vi "Valves_Widefield.vi"(1 "All Off?":bool, 2 "valve#":i32) -> ()   [LabVIEW 2012]
uses:
  <vilib>/DAQmx/create/channels.llb/DAQmx Create Channel (DO-Digital Output).vi
  <vilib>/DAQmx/write.llb/DAQmx Write (Digital 1D Bool NChan 1Samp 1Line).vi
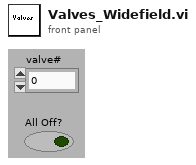
[diagram p1: front panel]
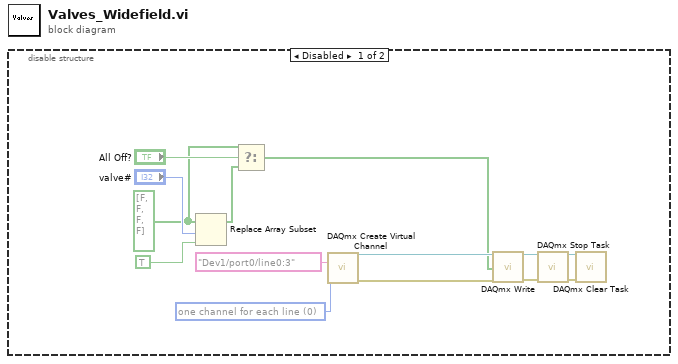
[diagram p0: block diagram]
diagram:
  n1 = disable-structure shown="Disabled" {
    frame Disabled {
      w3 = bool[] [FALSE, FALSE, FALSE, FALSE] ("port status")
      w7 = 0 items=["one channel for each line", "one channel for all lines"] ("line grouping")
      n2 = Replace Array Subset(array=w3, new element=TRUE ("new element/subarray"), index="valve#") -> (w2:bool[])
      n3 = Select(t=w3, s="All Off?", f=w2) -> (s? t:f=w1:bool[])
      n4 = call-poly <vilib>:"DAQmx Create Virtual Channel.vi"("lines"=tag "Dev1/port0/line0:3", "line grouping"=w7) -> ("task out"=w13:refnum<k21>, "error out"=w12:errorcluster)  [unwired: 3 in, 9 out]
      n5 = call-poly <vilib>:"DAQmx Write.vi"("task/channels in"=w13, "data"=w1, "error in"=w12) -> ("task out"=w11:refnum<k21>, "error out"=w10:errorcluster)  [unwired: 1 in, 10 out]
      n6 = call <vilib>:"DAQmx Stop Task.vi"("task/channels in"=w11, "error in"=w10) -> ("task out"=w9:refnum<k21>, "error out"=w8:errorcluster)  [unwired: 12 out]
      n7 = call <vilib>:"DAQmx Clear Task.vi"("task in"=w9, "error in"=w8) -> ()  [unwired: 14 out]
    }
    frame Enabled {
    }
  }
